vi "CameraKineticDEBUG.vi"() -> ()   [LabVIEW 2019]
uses:
  <vilib>/rvi/interface/nirviOpenFPGA/nirviOpenFPGA.xnode
  FPGA_bitfile/Jarvis_FPGATargetMacro_190515LV2017_nKk1DZ1Ci3E.lvbitx
  <vilib>/rvi/interface/nirviMethod/nirviMethod.xnode
  <vilib>/FPGAPlugInAG/Dynamic/niLvFpga_ConfigureFifo_Dynamic.vi
  <vilib>/rvi/errors/niLvFpgaMergeErrorWithErrorCode.vi
  <vilib>/rvi/interface/nirviReadWriteControl/nirviReadWriteControl.xnode
  NiFpgaLv.dll
  <vilib>/Utility/error.llb/Error Cluster From Error Code.vi
  <vilib>/rvi/interface/Simulation/niFpgaSimulationCallBeginRW.vi
  <vilib>/rvi/errors/niLvFpgaAdjustHostInterfaceError.vi
  <vilib>/rvi/interface/nirviCloseFPGA/nirviCloseFPGA.xnode
  <vilib>/FPGAPlugInAG/Dynamic/niLvFpga_Close_Dynamic.vi
  <vilib>/FPGAPlugInAG/PXI-7842R/niLvFpga_Open_PXI-7842R.vi
  <vilib>/rvi/interface/common/dynamic/niFpgaDynamicAddResources.vi
  VIs/Camera/CameraCoordsControl.ctl
  <userlib>/atmcd32d.llb/Error Code Enum typedef.ctl
panel:
  out "last 3":i32
  out "first 3":u32
  out "status 2":T1
  out "kinetic series data":i32[][][](array[numeric])
  in  "ion coords 2":T2={"Top :"=103.0, "Bottom :"=100.0, "Left :"=100.0, "Right :"=103.0}
  out "last 2":i32
  out "first 2":u32
  out "status":T1
  out "DLL error code 3":u32
  out "image size":cluster{"xpixels":i32, "ypixels":i32}
  out "DLL error code":u32
  out "error constant 2":errorcluster
  in  "ion coords":T2={"Top :"=103.0, "Bottom :"=100.0, "Left :"=100.0, "Right :"=103.0}
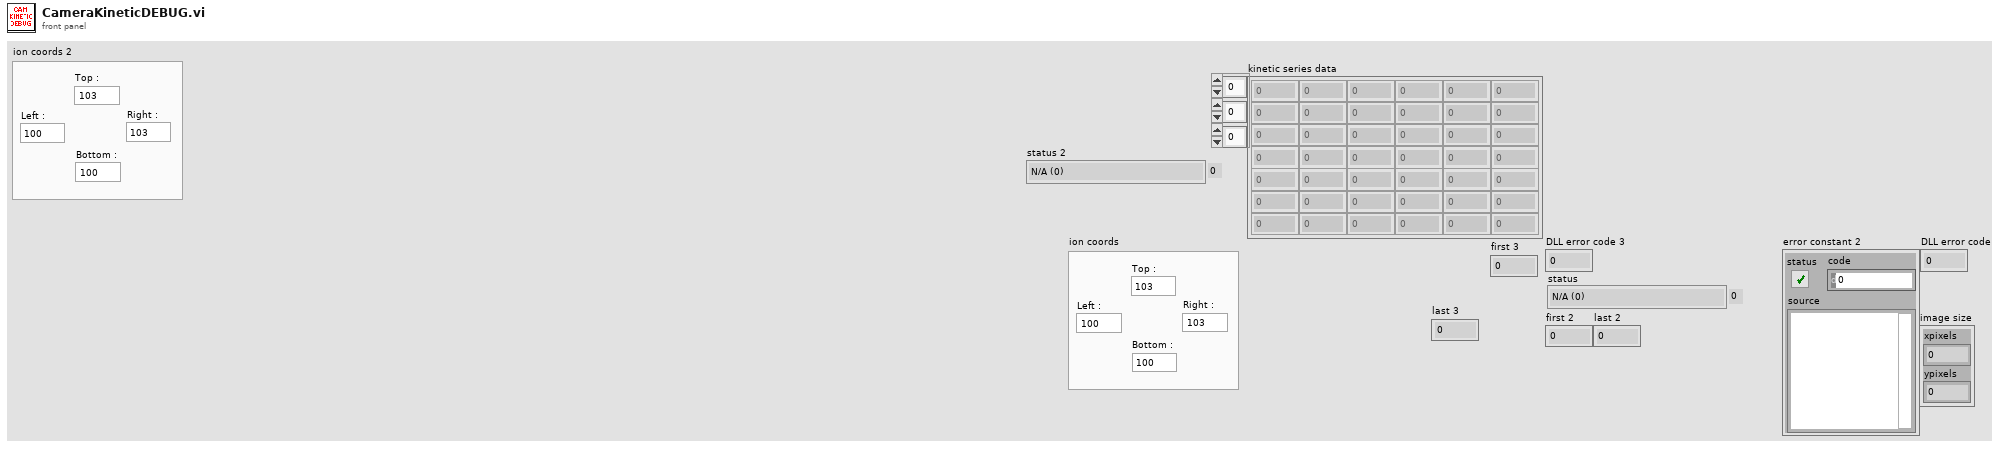
[diagram p1: front panel]
types:
  T1 = typedef "Error Code Enum typedef.ctl" = enum32{"N/A (0)", "DRV_ERROR_CODES", "DRV_SUCCESS", "DRV_VXDNOTINSTALLED", "DRV_ERROR_SCAN", "DRV_ERROR_CHECK_SUM", "DRV_ERROR_FILELOAD", "DRV_UNKNOWN_FUNC", "DRV_ERROR_VXD_INIT", "DRV_ERROR_ADDRESS", "DRV_ERROR_PAGELOCK", "DRV_ERROR_PAGEUNLOCK", "DRV_ERROR_BOARDTEST", "DRV_ERROR_ACK", "DRV_ERROR_UP_FIFO", "DRV_ERROR_PATTERN", "N/A (16)", "DRV_ACQUISITION_ERRORS", "DRV_ACQ_BUFFER", "DRV_ACQ_DOWNFIFO_FULL", "DRV_PROC_UNKONWN_INSTRUCTION", "DRV_ILLEGAL_OP_CODE", "DRV_KINETIC_TIME_NOT_MET", "DRV_ACCUM_TIME_NOT_MET", "DRV_NO_NEW_DATA", "N/A (25)", "DRV_SPOOLERROR", "N/A (27)", "N/A (28)", "N/A (29)", "N/A (30)", "N/A (31)", "N/A (32)", "DRV_TEMPERATURE_CODES", "DRV_TEMPERATURE_OFF", "DRV_TEMPERATURE_NOT_STABILIZED", "DRV_TEMPERATURE_STABILIZED", "DRV_TEMPERATURE_NOT_REACHED", "DRV_TEMPERATURE_OUT_RANGE", "DRV_TEMPERATURE_NOT_SUPPORTED", "DRV_TEMPERATURE_DRIFT", "N/A (41)", "N/A (42)", "N/A (43)", "N/A (44)", "N/A (45)", "N/A (46)", "N/A (47)", "N/A (48)", "DRV_GENERAL_ERRORS", "DRV_INVALID_AUX", "DRV_COF_NOTLOADED", "DRV_FPGAPROG", "DRV_FLEXERROR", "DRV_GPIBERROR", "N/A (55)", "N/A (56)", "N/A (57)", "N/A (58)", "N/A (59)", "N/A (60)", "N/A (61)", "N/A (62)", "N/A (63)", "DRV_DATATYPE", "DRV_DRIVER_ERRORS", "DRV_P1INVALID", "DRV_P2INVALID", "DRV_P3INVALID", "DRV_P4INVALID", "DRV_INIERROR", "DRV_COFERROR", "DRV_ACQUIRING", "DRV_IDLE", "DRV_TEMPCYCLE", "DRV_NOT_INITIALIZED", "DRV_P5INVALID", "DRV_P6INVALID", "DRV_INVALID_MODE", "DRV_INVALID_FILTER", "DRV_I2CERRORS", "DRV_I2CDEVNOTFOUND", "DRV_I2CTIMEOUT", "DRV_P7INVALID", "N/A (84)", "N/A (85)", "N/A (86)", "N/A (87)", "N/A (88)", "N/A (89)", "DRV_IOCERROR", "DRV_VRMVERSIONERROR"}
  T2 = typedef "CameraCoordsControl.ctl" = cluster{"Top :":dbl, "Bottom :":dbl, "Left :":dbl, "Right :":dbl}
  T3 = cluster{"Sequence Exposure Time (secs)":sgl, "# of kinetics":i32, "triggered?":bool}
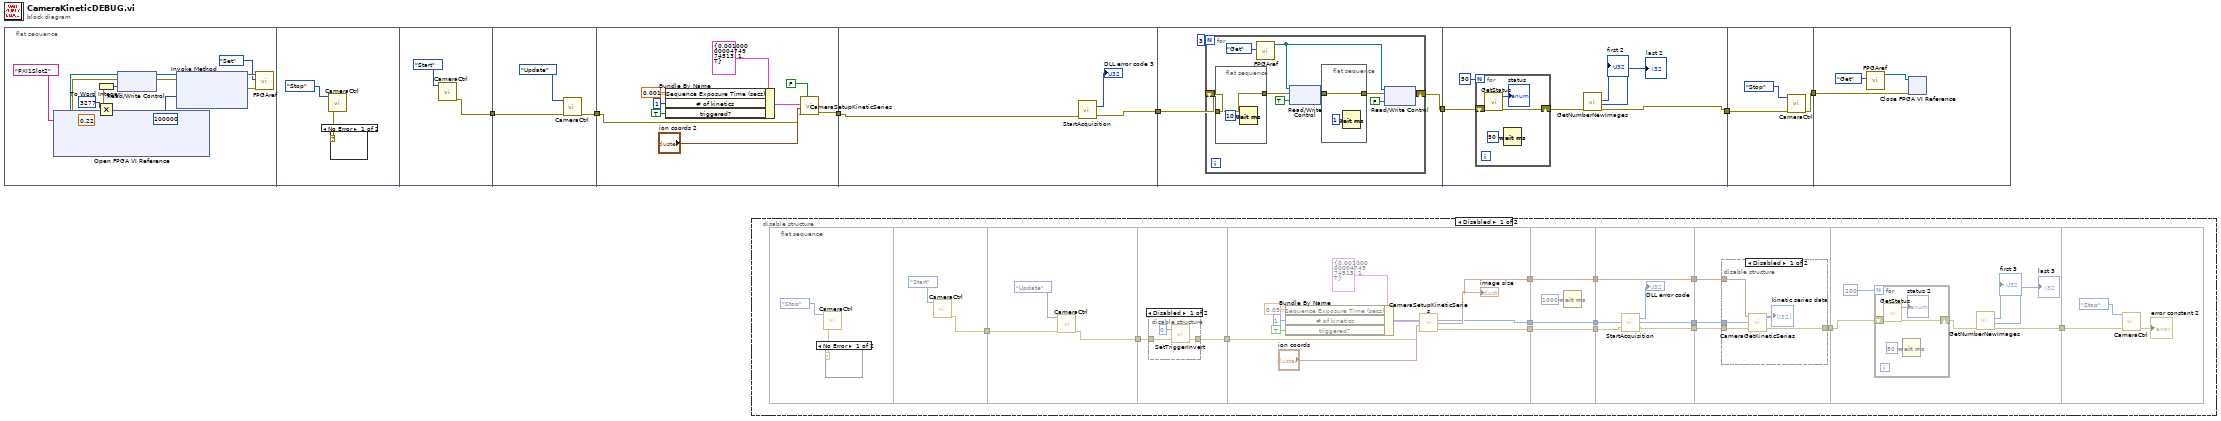
[diagram p0: block diagram]
diagram:
  n1 = flat-sequence {
    tunnel: [w23] -> w7
    tunnel: w7 -> [w26]
    tunnel: [w25] -> w6
    tunnel: w6 -> [w30]
    tunnel: [w29] -> w5
    tunnel: w5 -> [w37]
    tunnel: [w38] -> w3
    tunnel: w3 -> [w42]
    tunnel: [w41] -> w2
    tunnel: [w57] -> w4
    tunnel: w2 -> [w56]
    tunnel: w4 -> [w67]
    tunnel: [w66] -> w1
    tunnel: w1 -> [w69]
    frame #0 {
      n2 = xnode "Open FPGA VI Reference"("resource name"=tag "PXI1Slot2") -> ("FPGA VI Reference Out"=w15:refnum<k20>, "error out"=w13:errorcluster)  [unwired: 1 in]
      n3 = Multiply(x=3277, y=0.22) -> (x*y=w9:dbl)
      n4 = To Word Integer(number=w9) -> (16bit integer=w8:i16)
      n5 = xnode "Read/Write Control"("FPGA VI Reference In"=w15, "error in"=w13, "AO4 max"=w8) -> ("FPGA VI Reference Out"=w14:refnum<k20>, "error out"=w12:errorcluster)
      n6 = xnode "Invoke Method"("FPGA VI Reference In"=w14, "error in"=w12, "Requested Depth"=u32 100000) -> ("FPGA VI Reference Out"=w18:refnum<k20>, "error out"=w19:errorcluster)  [unwired: 1 out]
      n7 = call "FPGAref.vi"("error in"=w19, "Enum"=enum16{"Set", "Get"}."Set", "FPGA VI Reference Out"=w18) -> ()  [unwired: 3 in, 2 out]
    }
    frame #1 {
      n8 = call "CameraCtrl.vi"("Enum"=enum16{"Start", "Stop", "Acquire", "Update"}."Stop") -> ("error constant 2"=w22:errorcluster)  [unwired: 8 in, 2 out]
      n9 = case shown="No Error" w22 {
        frame No Error {
        }
        frame Error {
        }
      }
    }
    frame #2 {
      n10 = call "CameraCtrl.vi"("Enum"=enum16{"Start", "Stop", "Acquire", "Update"}."Start") -> ("error constant 2"=w23:errorcluster)  [unwired: 8 in, 2 out]
    }
    frame #3 {
      n11 = call "CameraCtrl.vi"("error constant"=w26, "Enum"=enum16{"Start", "Stop", "Acquire", "Update"}."Update") -> ("error constant 2"=w25:errorcluster)  [unwired: 7 in, 2 out]
    }
    frame #4 {
      n12 = Bundle By Name(cluster=T3 {"Sequence Exposure Time (secs)"=0.001, "# of kinetics"=1, "triggered?"=TRUE} ("kinetic series pars"), "Sequence Exposure Time (secs)"=sgl 0.001, "# of kinetics"=1, "triggered?"=TRUE) -> (w36:T3)
      n13 = call "CameraSetupKineticSeries.vi"("kinetic series pars"=w36, "subimage cluster"="ion coords 2", "error in (no error)"=w30, "EM adv"=FALSE) -> ("error out"=w29:errorcluster)  [unwired: 1 in, 2 out]
    }
    frame #5 {
      n14 = call <userlib>:"StartAcquisition.vi"("error in (no error)"=w37) -> ("error out"=w38:errorcluster, "DLL error code"=→"DLL error code 3":u32)  [unwired: 1 in]
    }
    frame #6 {
      n15 = for {
        N: 3 -> [_]
        shift-right: [w45] -> w41
        shift-left: w42 -> [w49]
        n16 = flat-sequence {
          tunnel: w49 -> [w53]
          tunnel: [w53] -> w48
          frame #0 {
            n17 = Wait (ms)(milliseconds to wait=u32 10) -> ()  [unwired: 1 out]
          }
        }
        n18 = call "FPGAref.vi"("Enum"=enum16{"Set", "Get"}."Get") -> ("FPGA VI Reference Out 2"=w44:refnum<k20>)  [unwired: 5 in, 1 out]
        n19 = xnode "Read/Write Control"("FPGA VI Reference In"=w44, "error in"=w48, "D22"=TRUE) -> ("error out"=w47:errorcluster)  [unwired: 1 out]
        n20 = flat-sequence {
          tunnel: w47 -> [w55]
          tunnel: [w55] -> w43
          frame #0 {
            n21 = Wait (ms)(milliseconds to wait=u32 1) -> ()  [unwired: 1 out]
          }
        }
        n22 = xnode "Read/Write Control"("FPGA VI Reference In"=w44, "error in"=w43, "D22"=FALSE) -> ("error out"=w45:errorcluster)  [unwired: 1 out]
      }
    }
    frame #7 {
      n23 = for {
        N: 50 -> [_]
        shift-right: [w64] -> w59
        shift-left: w56 -> [w65]
        n24 = call <userlib>:"GetStatus.vi"("error in (no error)"=w65) -> ("error out"=w64:errorcluster, "status"=→"status":T1)  [unwired: 2 in, 1 out]
        n25 = Wait (ms)(milliseconds to wait=u32 50) -> ()  [unwired: 1 out]
      }
      n26 = call <userlib>:"GetNumberNewImages.vi"("error in (no error)"=w59) -> ("error out"=w57:errorcluster, "last"=→"last 2":i32, "first"=→"first 2":u32)  [unwired: 3 in, 1 out]
    }
    frame #8 {
      n27 = call "CameraCtrl.vi"("error constant"=w67, "Enum"=enum16{"Start", "Stop", "Acquire", "Update"}."Stop") -> ("error constant 2"=w66:errorcluster)  [unwired: 7 in, 2 out]
    }
    frame #9 {
      n28 = call "FPGAref.vi"("Enum"=enum16{"Set", "Get"}."Get") -> ("FPGA VI Reference Out 2"=w70:refnum<k20>)  [unwired: 5 in, 1 out]
      n29 = xnode "Close FPGA VI Reference"("FPGA VI Reference In"=w70, "error in"=w69) -> ()  [unwired: 1 out]
    }
  }
  n30 = disable-structure shown="Disabled" {
    frame Disabled {
      n31 = flat-sequence {
        tunnel: [w88] -> w85
        tunnel: w85 -> [w91]
        tunnel: [w90] -> w84
        tunnel: w84 -> [w94]
        tunnel: [w93] -> w83
        tunnel: w83 -> [w101]
        tunnel: [w100] -> w82
        tunnel: [w99] -> w81
        tunnel: [w98] -> w80
        tunnel: w82 -> [w110]
        tunnel: [w110] -> w79
        tunnel: [w108] -> w78
        tunnel: w81 -> [w108]
        tunnel: w80 -> [w107]
        tunnel: [w107] -> w77
        tunnel: w79 -> [w115]
        tunnel: [w113] -> w76
        tunnel: [w112] -> w75
        tunnel: w78 -> [w112]
        tunnel: w77 -> [w111]
        tunnel: [w111] -> w74
        tunnel: [w118] -> w73
        tunnel: w76 -> [w119]
        tunnel: w75 -> [w117]
        tunnel: w74 -> [w116]
        tunnel: w73 -> [w129]
        tunnel: [w125] -> w72
        tunnel: w72 -> [w136]
        frame #0 {
          n32 = call "CameraCtrl.vi"("Enum"=enum16{"Start", "Stop", "Acquire", "Update"}."Stop") -> ("error constant 2"=w87:errorcluster)  [unwired: 8 in, 2 out]
          n33 = case shown="No Error" w87 {
            frame No Error {
            }
            frame Error {
            }
          }
        }
        frame #1 {
          n34 = call "CameraCtrl.vi"("Enum"=enum16{"Start", "Stop", "Acquire", "Update"}."Start") -> ("error constant 2"=w88:errorcluster)  [unwired: 8 in, 2 out]
        }
        frame #2 {
          n35 = call "CameraCtrl.vi"("error constant"=w91, "Enum"=enum16{"Start", "Stop", "Acquire", "Update"}."Update") -> ("error constant 2"=w90:errorcluster)  [unwired: 7 in, 2 out]
        }
        frame #3 {
          n36 = disable-structure shown="Disabled" {
            disable-tunnel: w94 -> [w97 _]
            disable-tunnel: [w96 _] -> w93
            frame Disabled {
              n37 = call <userlib>:"SetTriggerInvert.vi"("error in (no error)"=w97, "mode"=0) -> ("error out"=w96:errorcluster)  [unwired: 1 out]
            }
            frame Enabled {
            }
          }
        }
        frame #4 {
          w98 = 1 ("# of kinetics")
          n38 = Bundle By Name(cluster=T3 {"Sequence Exposure Time (secs)"=0.001, "# of kinetics"=1, "triggered?"=TRUE} ("kinetic series pars"), "Sequence Exposure Time (secs)"=sgl 0.05, "# of kinetics"=w98, "triggered?"=TRUE) -> (w106:T3)
          n39 = call "CameraSetupKineticSeries.vi"("kinetic series pars"=w106, "subimage cluster"="ion coords", "error in (no error)"=w101) -> ("image size"=w99:cluster{"xpixels":i32, "ypixels":i32}, "error out"=w100:errorcluster)  [unwired: 2 in, 1 out]
          "image size" <- w99
        }
        frame #5 {
          n40 = Wait (ms)(milliseconds to wait=u32 1000) -> ()  [unwired: 1 out]
        }
        frame #6 {
          n41 = call <userlib>:"StartAcquisition.vi"("error in (no error)"=w115) -> ("error out"=w113:errorcluster, "DLL error code"=→"DLL error code":u32)  [unwired: 1 in]
        }
        frame #7 {
          n42 = disable-structure shown="Disabled" {
            disable-tunnel: w119 -> [w124 _]
            disable-tunnel: [w123 _] -> w118
            disable-tunnel: w117 -> [w122 _]
            disable-tunnel: w116 -> [w121 _]
            frame Disabled {
              n43 = call "CameraGetKineticSeries.vi"("error out 2"=w124, "# of kinetics"=w121, "image size"=w122) -> ("error out"=w123:errorcluster, "kinetic series data"=→"kinetic series data":i32[][][])  [unwired: 1 in]
            }
            frame Enabled {
            }
          }
        }
        frame #8 {
          n44 = for {
            N: 200 -> [_]
            shift-right: [w133] -> w126
            shift-left: w129 -> [w134]
            n45 = call <userlib>:"GetStatus.vi"("error in (no error)"=w134) -> ("error out"=w133:errorcluster, "status"=→"status 2":T1)  [unwired: 2 in, 1 out]
            n46 = Wait (ms)(milliseconds to wait=u32 50) -> ()  [unwired: 1 out]
          }
          n47 = call <userlib>:"GetNumberNewImages.vi"("error in (no error)"=w126) -> ("error out"=w125:errorcluster, "last"=→"last 3":i32, "first"=→"first 3":u32)  [unwired: 3 in, 1 out]
        }
        frame #9 {
          n48 = call "CameraCtrl.vi"("error constant"=w136, "Enum"=enum16{"Start", "Stop", "Acquire", "Update"}."Stop") -> ("error constant 2"=→"error constant 2":errorcluster)  [unwired: 7 in, 2 out]
        }
      }
    }
    frame Enabled {
    }
  }
